vi "SPOL_ops_mode.vi"() -> ()   [LabVIEW 2012]
doc: "Use this template to build a producer/consumer design pattern with events to produce queue items. Use this design pattern instead of the User Interface Event Handler pattern for user interfaces when you want to execute code asynchronously in response to an event without slowing the user interface responsiveness."
panel:
  out "Signal Generator Status":T1={"Frequency (GHz)"=2809000000.0, "RF Power (dBm)"=-120.0, "RF Power"=FALSE} {"RF Power (dBm)" format="%.2g"}
  out "Error out":errorcluster
  out "70 Verified":bool
  out "Xmit Enable":bool
  out "121 Verified":bool
  out "Inside Noise Box":bool
  out "Outside Noise Box":bool
  out "ATE Switch Status":T2
  in  "WG3 MS":bool
  out "WG3":bool
  in  "WG2 MS":bool
  out "WG2":bool
  in  "WG1 MS":bool
  out "WG1":bool
  in  "WG5 ANT":bool
  out "WG5":bool
  in  "WG4 ANT":bool
  out "WG4":bool
  # "SPOL OPS Mode"
  # "All ATE switches OPEN\n121 and 70 dB attenuaters active\nNoise sources disabled\nTransmitter enabled\nWave guide switches in ops mode\nTest pulse enabled at -20dBm"
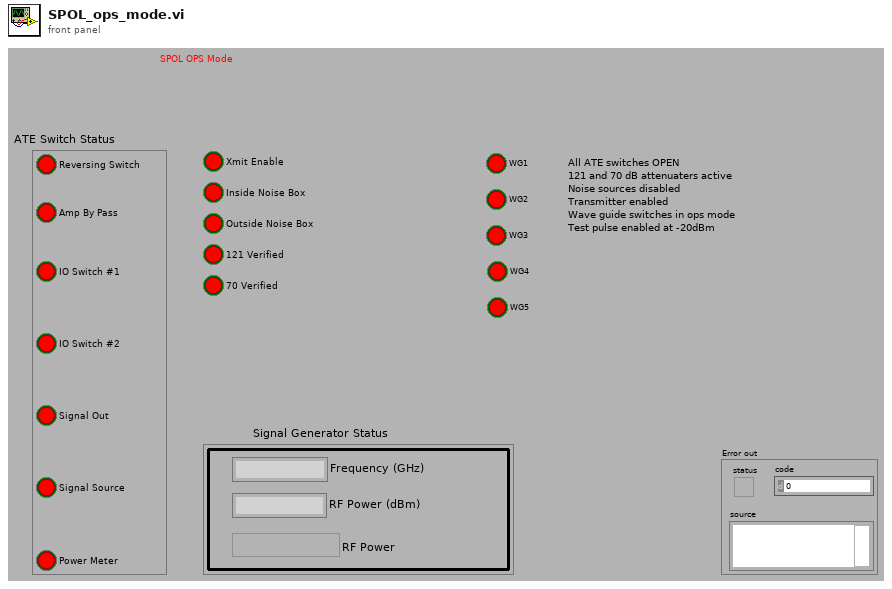
[diagram p1: front panel]
types:
  T1 = cluster{"Frequency (GHz)":dbl, "RF Power (dBm)":dbl, "RF Power":bool}
  T2 = cluster{"Reversing Switch ":bool, "IO Switch #1":bool, "IO Switch #2":bool, "Signal Out":bool, "Signal Source":bool, "Power Meter":bool, "Amp By Pass":bool}
  T3 = cluster{"Frequency (GHz)":dbl, "RF Power (dBm)":dbl, "RF ON/OFF":bool}
  T4 = cluster{"Reversing Switch":enum16{"Normal Function", "Reversing Function"}, "IO Switch #1 Input":enum16{"NONE", "AHR (J2)", "Splitter", "Signal Out Switch (S3)", "Reversing Switch"}, "IO Switch #1 Output":enum16{"NONE", "AHR (J2)", "Delay Device (S4)", "Power Meter Switch (S5)", "Reversing Switch"}, "IO Switch #2 Input":enum16{"NONE", "AVR (J3)", "Splitter", "Signal Out Switch (S3)", " 2W Term (TM1)", "Reversing Switch"}, "IO Switch #2 Output":enum16{"NONE", "AVR (J3)", "Signal Out Switch (S3)", "Power Meter Switch (S5)", "Reversing Switch", "2W Term (TM1)"}, "Signal Out Input":enum16{"NONE", "Amp Bypass Switch (S6)", "IO Switch #1 (S1)", "IO Switch #2 (S2)", "2W Term (TM3)"}, "Signal Out Output":enum16{"NONE", "2 Watt Term (TM3)", "Splitter", "Power Meter Switch (S5)"}, "Signal Source Input":enum16{"NONE", "Delay Device", "Signal Generator (J7)", "Inside Noise Box NF (J5)", "2W Term (TM3)"}, "Signal Source Output":enum16{"NONE", "Amp Bypass Switch", "Test Pulse Generator", "Power Meter Switch (S5)"}, "Power Meter Switch Input":enum16{"NONE", "IO Switch #1 (S1)", "Signal Source Switch (S4)", "Signal Out Switch (S3)", "IO Switch #2 (S2)", "TXH-TXV Switch (J8)"}, "Pouer Meter Switch Output":enum16{"NONE", "Power Meter (J6)"}, "Amplifier Switch":enum16{"Bypass Amp", "Include Amp"}}
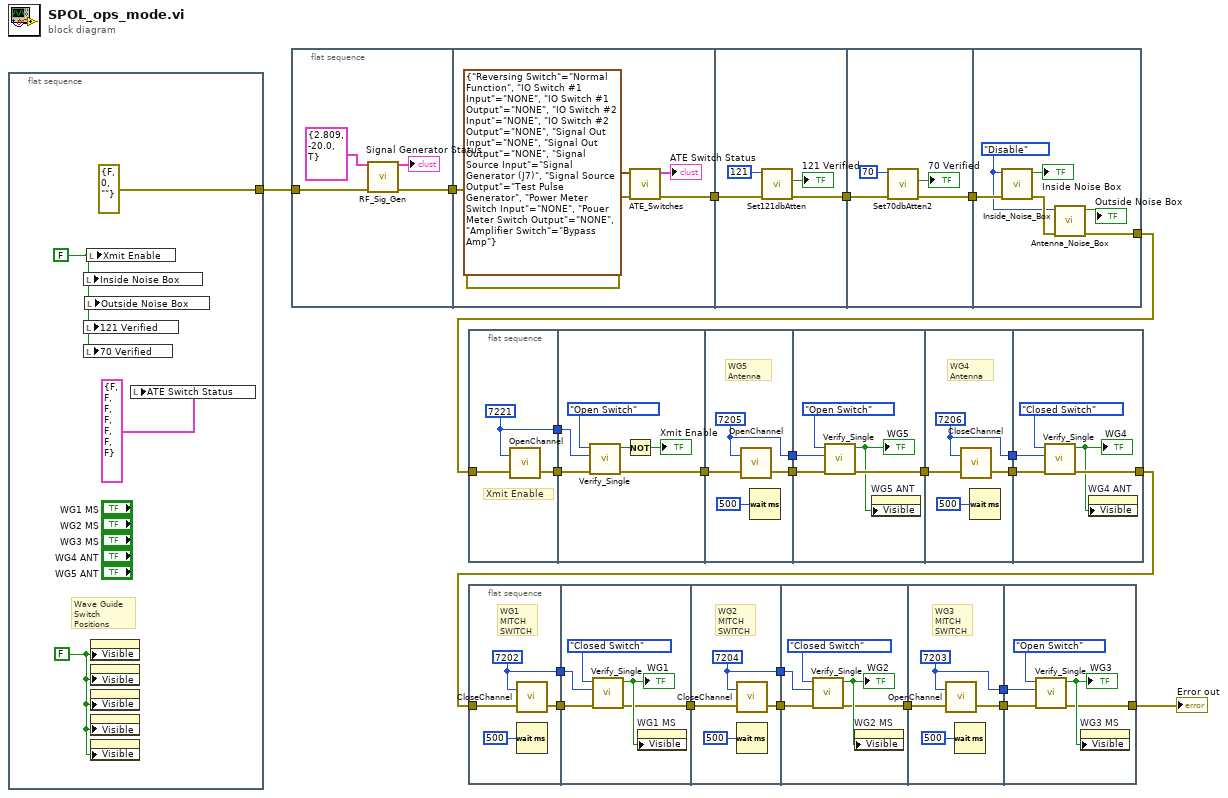
[diagram p0: block diagram]
diagram:
  n1 = flat-sequence {
    tunnel: [errorcluster {"status"=FALSE, "code"=0, "source"=""} ("error in")] -> w1
    frame #0 {
      w25 = FALSE ("121 Verified")
      w27 = FALSE ("Visible")
      # "Wave Guide\nSwitch\nPositions"
      n2 = local write "Inside Noise Box"(w25) -> ()
      n3 = local write "121 Verified"(w25) -> ()
      n4 = local write "70 Verified"(w25) -> ()
      n5 = local write "Outside Noise Box"(w25) -> ()
      n6 = local write "Xmit Enable"(w25) -> ()
      n7 = property on="WG1 MS" class="Bool"("Visible"=w27) -> ()  [unwired: 2 in, 2 out]
      n8 = property on="WG2 MS" class="Bool"("Visible"=w27) -> ()  [unwired: 2 in, 2 out]
      n9 = property on="WG3 MS" class="Bool"("Visible"=w27) -> ()  [unwired: 2 in, 2 out]
      n10 = property on="WG4 ANT" class="Bool"("Visible"=w27) -> ()  [unwired: 2 in, 2 out]
      n11 = property on="WG5 ANT" class="Bool"("Visible"=w27) -> ()  [unwired: 2 in, 2 out]
      n12 = local write "ATE Switch Status"(T2 {"Reversing Switch "=FALSE, "IO Switch #1"=FALSE, "IO Switch #2"=FALSE, "Signal Out"=FALSE, "Signal Source"=FALSE, "Power Meter"=FALSE, "Amp By Pass"=FALSE} ("ATE Switch Status")) -> ()
    }
  }
  n13 = flat-sequence {
    tunnel: [w31] -> w24
    tunnel: w1 -> [w30]
    tunnel: [w34] -> w23
    tunnel: w24 -> [w35]
    tunnel: w23 -> [w40]
    tunnel: [w39] -> w22
    tunnel: w22 -> [w44]
    tunnel: [w42] -> w21
    tunnel: w21 -> [w50]
    tunnel: [w45] -> w3
    frame #0 {
      n14 = call "RF_Sig_Gen.vi"("Signal Generator Control"=T3 {"Frequency (GHz)"=2.809, "RF Power (dBm)"=-20.0, "RF ON/OFF"=TRUE}, "error in"=w30) -> ("Signal Generator Status"=→"Signal Generator Status":T1, "Sig Gen Errors"=w31:errorcluster)  [unwired: 12 in]
    }
    frame #1 {
      n15 = call "ATE_Switches.vi"("error in"=w35, "ATE Switches"=T4 {"Reversing Switch"=enum."Normal Function", "IO Switch #1 Input"=enum."NONE", "IO Switch #1 Output"=enum."NONE", "IO Switch #2 Input"=enum."NONE", "IO Switch #2 Output"=enum."NONE", "Signal Out Input"=enum."NONE", "Signal Out Output"=enum."NONE", "Signal Source Input"=enum."Signal Generator (J7)", "Signal Source Output"=enum."Test Pulse Generator", "Power Meter Switch Input"=enum."NONE", "Pouer Meter Switch Output"=enum."NONE", "Amplifier Switch"=enum."Bypass Amp"}) -> ("Switch Errors"=w34:errorcluster, "ATE Switch Status"=→"ATE Switch Status":T2)  [unwired: 8 in]
    }
    frame #2 {
      n16 = call "Set121dbAtten.vi"("error in (no error)"=w40, "Attenuation (dB)"=121) -> ("error out"=w39:errorcluster, "Verfied"=→"121 Verified":bool)  [unwired: 7 in, 1 out]
    }
    frame #3 {
      n17 = call "Set70dbAtten2.vi"("error in (no error)"=w44, "Attenuation (dB)"=70) -> ("error out"=w42:errorcluster, "Verfied"=→"70 Verified":bool)  [unwired: 7 in, 1 out]
    }
    frame #4 {
      w46 = enum16{"Disable", "Enable"}."Disable" ("Noise Switch Function")
      n18 = call "Inside_Noise_Box.vi"("error in"=w50, "Noise Switch Function"=w46) -> ("error out"=w49:errorcluster, "Verfied"=→"Inside Noise Box":bool)  [unwired: 8 in]
      n19 = call "Antenna_Noise_Box.vi"("error in"=w49, "Noise Switch Function"=w46) -> ("error out"=w45:errorcluster, "Verfied"=→"Outside Noise Box":bool)  [unwired: 8 in]
    }
  }
  n20 = flat-sequence {
    tunnel: [w53] -> w5
    tunnel: [w52] -> w4
    tunnel: w3 -> [w51]
    tunnel: [w58] -> w20
    tunnel: w5 -> [w57]
    tunnel: w4 -> [w56]
    tunnel: w20 -> [w63]
    tunnel: [w62] -> w19
    tunnel: [w61] -> w18
    tunnel: [w65] -> w17
    tunnel: w19 -> [w67]
    tunnel: w18 -> [w66]
    tunnel: [w70] -> w16
    tunnel: w17 -> [w72]
    tunnel: [w69] -> w15
    tunnel: w16 -> [w76]
    tunnel: w15 -> [w75]
    tunnel: [w74] -> w6
    frame #0 {
      w52 = 7221
      # "Xmit Enable"
      n21 = call "OpenChannel.vi"("error in (no error)"=w51, "Channel ID"=w52) -> ("error out"=w53:errorcluster)  [unwired: 1 in]
    }
    frame #1 {
      n22 = call "Verify_Single.vi"("error in"=w57, "Switch ID"=w56, "Switch Functin"=enum16{"Open Switch", "Closed Switch"}."Open Switch") -> ("Error out"=w58:errorcluster, "Verfied"=w55:bool)  [unwired: 7 in]
      n23 = Not(x=w55) -> (.not. x?=→"Xmit Enable":bool)
    }
    frame #2 {
      w61 = 7205
      # "WG5\nAntenna"
      n24 = call "OpenChannel.vi"("error in (no error)"=w63, "Channel ID"=w61) -> ("error out"=w62:errorcluster)  [unwired: 1 in]
      n25 = Wait (ms)(milliseconds to wait=u32 500) -> ()  [unwired: 1 out]
    }
    frame #3 {
      n26 = call "Verify_Single.vi"("error in"=w67, "Switch ID"=w66, "Switch Functin"=enum16{"Open Switch", "Closed Switch"}."Open Switch") -> ("Error out"=w65:errorcluster, "Verfied"=w64:bool)  [unwired: 7 in]
      "WG5" <- w64
      n27 = property on="WG5 ANT" class="Bool"("Visible"=w64) -> ()  [unwired: 2 in, 2 out]
    }
    frame #4 {
      w69 = 7206
      # "WG4\nAntenna"
      n28 = call "CloseChannel.vi"("error in (no error)"=w72, "Channel ID"=w69) -> ("error out"=w70:errorcluster)  [unwired: 1 in]
      n29 = Wait (ms)(milliseconds to wait=u32 500) -> ()  [unwired: 1 out]
    }
    frame #5 {
      n30 = call "Verify_Single.vi"("error in"=w76, "Switch ID"=w75, "Switch Functin"=enum16{"Open Switch", "Closed Switch"}."Closed Switch") -> ("Error out"=w74:errorcluster, "Verfied"=w73:bool)  [unwired: 7 in]
      "WG4" <- w73
      n31 = property on="WG4 ANT" class="Bool"("Visible"=w73) -> ()  [unwired: 2 in, 2 out]
    }
  }
  n32 = flat-sequence {
    tunnel: [w80] -> w14
    tunnel: [w79] -> w13
    tunnel: w6 -> [w78]
    tunnel: w14 -> [w85]
    tunnel: [w83] -> w12
    tunnel: w13 -> [w82]
    tunnel: w12 -> [w89]
    tunnel: [w88] -> w11
    tunnel: [w87] -> w10
    tunnel: w11 -> [w94]
    tunnel: w10 -> [w93]
    tunnel: [w91] -> w9
    tunnel: w9 -> [w98]
    tunnel: [w97] -> w8
    tunnel: [w96] -> w7
    tunnel: w8 -> [w102]
    tunnel: w7 -> [w103]
    tunnel: [w100] -> w2
    frame #0 {
      w79 = 7202
      # "WG1\nMITCH\nSWITCH"
      n33 = call "CloseChannel.vi"("error in (no error)"=w78, "Channel ID"=w79) -> ("error out"=w80:errorcluster)  [unwired: 1 in]
      n34 = Wait (ms)(milliseconds to wait=u32 500) -> ()  [unwired: 1 out]
    }
    frame #1 {
      n35 = call "Verify_Single.vi"("error in"=w85, "Switch ID"=w82, "Switch Functin"=enum16{"Open Switch", "Closed Switch"}."Closed Switch") -> ("Error out"=w83:errorcluster, "Verfied"=w84:bool)  [unwired: 7 in]
      "WG1" <- w84
      n36 = property on="WG1 MS" class="Bool"("Visible"=w84) -> ()  [unwired: 2 in, 2 out]
    }
    frame #2 {
      w87 = 7204
      # "WG2\nMITCH\nSWITCH"
      n37 = call "CloseChannel.vi"("error in (no error)"=w89, "Channel ID"=w87) -> ("error out"=w88:errorcluster)  [unwired: 1 in]
      n38 = Wait (ms)(milliseconds to wait=u32 500) -> ()  [unwired: 1 out]
    }
    frame #3 {
      n39 = call "Verify_Single.vi"("error in"=w94, "Switch ID"=w93, "Switch Functin"=enum16{"Open Switch", "Closed Switch"}."Closed Switch") -> ("Error out"=w91:errorcluster, "Verfied"=w92:bool)  [unwired: 7 in]
      "WG2" <- w92
      n40 = property on="WG2 MS" class="Bool"("Visible"=w92) -> ()  [unwired: 2 in, 2 out]
    }
    frame #4 {
      w97 = 7203
      # "WG3\nMITCH\nSWITCH"
      n41 = call "OpenChannel.vi"("error in (no error)"=w98, "Channel ID"=w97) -> ("error out"=w96:errorcluster)  [unwired: 1 in]
      n42 = Wait (ms)(milliseconds to wait=u32 500) -> ()  [unwired: 1 out]
    }
    frame #5 {
      n43 = call "Verify_Single.vi"("error in"=w103, "Switch ID"=w102, "Switch Functin"=enum16{"Open Switch", "Closed Switch"}."Open Switch") -> ("Error out"=w100:errorcluster, "Verfied"=w101:bool)  [unwired: 7 in]
      "WG3" <- w101
      n44 = property on="WG3 MS" class="Bool"("Visible"=w101) -> ()  [unwired: 2 in, 2 out]
    }
  }
  "Error out" <- w2
